vi "ForceShutdown.vi"() -> ()   [LabVIEW 2013]
uses:
  ATMCD32D.dll
panel:
  out "return type":i32
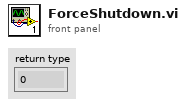
[diagram p1: front panel]
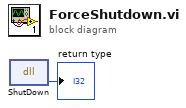
[diagram p0: block diagram]
diagram:
  n1 = dll-call lib="atmcd32d.dll" fn="ShutDown"() -> ("return type"=→"return type":i32)  [unwired: 3 in, 2 out]
